vi "WriteOnshapeAngle.vi"(8 "Angle2In":dbl, 9 "Angle1In":dbl, 10 "IDs":T1={"did"="37b1ffe826404682316d4eb0", "wid"="5d55043850c7dcf86f882f4b", "eid"="763f42ab39165e5d749d00a9"}) -> ()   [LabVIEW 2022 SP3]
uses:
  _SubVI/HTTPComm.ctl
panel:
  in  "error in":errorcluster
  out "error out":errorcluster
  out "payload":string
  out "Comm":T2={"url"="https://rogers.onshape.com/api/partstudios/d/78f5bf641b1754cc5a2885a6/w/2816a0ac3f158e698c5324a2/e/990ec2d1208dce12e8c8d73d/sketches?", "sent headers"="Accept: application/json\r\nAuthorization: On 5WRzTWmAmwc94xTxHfKZAg5i:HmacSHA256:lDyQC1x2JlGNCtdzVGE5L8N41PUpGQIlxBBiesg5jjs=\r\nContent-Type: application/json\r\nDate: Thu, 16 Apr 2020 23:19:12 GMT\r\nOn-Nonce: nlS7Y9rr4jS35A8DK9B3OToU\r\nUser_agent: Onshape Python Sample App", "sent body"="", "headers"="HTTP/1.1 200 OK\r\nServer: nginx\r\nDate: Thu, 16 Apr 2020 23:19:12 GMT\r\nContent-Type: application/json;charset=UTF-8;qs=0.9\r\nContent-Length: 2372\r\nConnection: keep-alive\r\nVary: Accept-Encoding\r\nOn-Version: 1.111.25149.0c1f2eb083aa\r\nOn-Request-Id: a78cc699fde7b461387b36e3\r\nDeprecation: version=UNDEFINED, message=\"You specified mediatype application/json;charset=UTF-8;qs=0.9 and this endpoint will currently accept application/vnd.onshape.v1+json;charset=UTF-8;qs=0.1. Please consider updating to the latest version by specifying application/vnd.onshape.v1+json;charset=UTF-8;qs=0.1 within the Accept header.\r\nSet-Cookie: _u=webservice-3e25a82e; Path=/; Secure; HttpOnly;\r\nX-Frame-Options: SAMEORIGIN\r\nStrict-Transport-Security: max-age=31536000; includeSubDomains\r\nX-Content-Type-Options: nosniff\r\nX-XSS-Protection: 1; mode=block\r\nContent-Security-Policy-Report-Only: object-src 'self' https://embedwistia-a.akamaihd.net; report-uri /api/csp\r\n\r\n", "body"="{\n  \"sketches\" : [ {\n    \"sketch\" : \"Sketch 1\",\n    \"featureId\" : \"FbqM6rYzUBbMRp8_0\",\n    \"transformMatrix\" : [ 1.0, 0.0, 0.0, 0.0, 0.0, 1.0, 0.0, 0.0, 0.0, 0.0, 1.0, 0.0, 0.0, 0.0, 0.0, 1.0 ],\n    \"featuresUsed\" : [ ],\n    \"geomEntities\" : [ {\n      \"id\" : \"C471k0qsEi0Q.start\",\n      \"entityType\" : \"point\",\n      \"point\" : [ 0.017283352091908455, -0.007151731755584478 ]\n    }, {\n      \"id\" : \"C471k0qsEi0Q.end\",\n      \"entityType\" : \"point\",\n      \"point\" : [ -0.04529430344700813, 0.05423396825790405 ]\n    }, {\n      \"id\" : \"C471k0qsEi0Q.0.internal\",\n      \"entityType\" : \"point\",\n      \"point\" : [ 0.017283352091908455, -0.007151731755584478 ]\n    }, {\n      \"id\" : \"C471k0qsEi0Q.1.internal\",\n      \"entityType\" : \"point\",\n      \"point\" : [ 0.05095608904957771, 0.022945139557123184 ]\n    }, {\n      \"id\" : \"C471k0qsEi0Q.2.internal\",\n      \"entityType\" : \"point\",\n      \"point\" : [ 0.02443508431315422, 0.05780983343720436 ]\n    }, {\n      \"id\" : \"C471k0qsEi0Q.3.internal\",\n      \"entityType\" : \"point\",\n      \"point\" : [ -0.018177319318056107, 0.039334528148174286 ]\n    }, {\n      \"id\" : \"C471k0qsEi0Q.4.internal\",\n      \"entityType\" : \"point\",\n      \"point\" : [ -0.04529430344700813, 0.05423396825790405 ]\n    }, {\n      \"id\" : \"C471k0qsEi0Q.startDerivative\",\n      \"entityType\" : \"point\",\n      \"point\" : [ 0.03353424071398461, 8.902966705931049E-4 ],\n      \"isConstruction\" : true\n    }, {\n      \"id\" : \"C471k0qsEi0Q.endDerivative\",\n      \"entityType\" : \"point\",\n      \"point\" : [ -0.0368764138795279, 0.04584760236142172 ],\n      \"isConstruction\" : true\n    }, {\n      \"id\" : \"C471k0qsEi0Q\",\n      \"entityType\" : \"interpolatedSplineSegment\",\n      \"periodic\" : false,\n      \"startHandle\" : [ 0.03353424071398461, 8.902966705931043E-4 ],\n      \"endHandle\" : [ -0.03687641387952791, 0.045847602361421734 ],\n      \"startDerivative\" : [ 0.18655982097041743, 0.0923222980796617 ],\n      \"endDerivative\" : [ -0.1167534466674709, 0.11631622339302505 ],\n      \"interpolationPoints\" : [ [ 0.017283352091908455, -0.007151731755584478 ], [ 0.05095608904957771, 0.022945139557123184 ], [ 0.02443508431315422, 0.05780983343720436 ], [ -0.018177319318056107, 0.039334528148174286 ], [ -0.04529430344700813, 0.05423396825790405 ] ],\n      \"startParameter\" : 0.0,\n      \"endParameter\" : 1.0,\n      \"endPointIds\" : [ \"C471k0qsEi0Q.start\", \"C471k0qsEi0Q.end\" ]\n    } ]\n  } ]\n}", "Sent"="get https://rogers.onshape.com/api/partstudios/d/78f5bf641b1754cc5a2885a6/w/2816a0ac3f158e698c5324a2/e/990ec2d1208dce12e8c8d73d/sketches? \n\nAccept: application/json\r\nAuthorization: On 5WRzTWmAmwc94xTxHfKZAg5i:HmacSHA256:lDyQC1x2JlGNCtdzVGE5L8N41PUpGQIlxBBiesg5jjs=\r\nContent-Type: application/json\r\nDate: Thu, 16 Apr 2020 23:19:12 GMT\r\nOn-Nonce: nlS7Y9rr4jS35A8DK9B3OToU\r\nUser_agent: Onshape Python Sample App\n\n", "Received"="HTTP/1.1 200 OK\r\nServer: nginx\r\nDate: Thu, 16 Apr 2020 23:19:12 GMT\r\nContent-Type: application/json;charset=UTF-8;qs=0.9\r\nContent-Length: 2372\r\nConnection: keep-alive\r\nVary: Accept-Encoding\r\nOn-Version: 1.111.25149.0c1f2eb083aa\r\nOn-Request-Id: a78cc699fde7b461387b36e3\r\nDeprecation: version=UNDEFINED, message=\"You specified mediatype application/json;charset=UTF-8;qs=0.9 and this endpoint will currently accept application/vnd.onshape.v1+json;charset=UTF-8;qs=0.1. Please consider updating to the latest version by specifying application/vnd.onshape.v1+json;charset=UTF-8;qs=0.1 within the Accept header.\r\nSet-Cookie: _u=webservice-3e25a82e; Path=/; Secure; HttpOnly;\r\nX-Frame-Options: SAMEORIGIN\r\nStrict-Transport-Security: max-age=31536000; includeSubDomains\r\nX-Content-Type-Options: nosniff\r\nX-XSS-Protection: 1; mode=block\r\nContent-Security-Policy-Report-Only: object-src 'self' https://embedwistia-a.akamaihd.net; report-uri /api/csp\r\n\r\n\n\n{\n  \"sketches\" : [ {\n    \"sketch\" : \"Sketch 1\",\n    \"featureId\" : \"FbqM6rYzUBbMRp8_0\",\n    \"transformMatrix\" : [ 1.0, 0.0, 0.0, 0.0, 0.0, 1.0, 0.0, 0.0, 0.0, 0.0, 1.0, 0.0, 0.0, 0.0, 0.0, 1.0 ],\n    \"featuresUsed\" : [ ],\n    \"geomEntities\" : [ {\n      \"id\" : \"C471k0qsEi0Q.start\",\n      \"entityType\" : \"point\",\n      \"point\" : [ 0.017283352091908455, -0.007151731755584478 ]\n    }, {\n      \"id\" : \"C471k0qsEi0Q.end\",\n      \"entityType\" : \"point\",\n      \"point\" : [ -0.04529430344700813, 0.05423396825790405 ]\n    }, {\n      \"id\" : \"C471k0qsEi0Q.0.internal\",\n      \"entityType\" : \"point\",\n      \"point\" : [ 0.017283352091908455, -0.007151731755584478 ]\n    }, {\n      \"id\" : \"C471k0qsEi0Q.1.internal\",\n      \"entityType\" : \"point\",\n      \"point\" : [ 0.05095608904957771, 0.022945139557123184 ]\n    }, {\n      \"id\" : \"C471k0qsEi0Q.2.internal\",\n      \"entityType\" : \"point\",\n      \"point\" : [ 0.02443508431315422, 0.05780983343720436 ]\n    }, {\n      \"id\" : \"C471k0qsEi0Q.3.internal\",\n      \"entityType\" : \"point\",\n      \"point\" : [ -0.018177319318056107, 0.039334528148174286 ]\n    }, {\n      \"id\" : \"C471k0qsEi0Q.4.internal\",\n      \"entityType\" : \"point\",\n      \"point\" : [ -0.04529430344700813, 0.05423396825790405 ]\n    }, {\n      \"id\" : \"C471k0qsEi0Q.startDerivative\",\n      \"entityType\" : \"point\",\n      \"point\" : [ 0.03353424071398461, 8.902966705931049E-4 ],\n      \"isConstruction\" : true\n    }, {\n      \"id\" : \"C471k0qsEi0Q.endDerivative\",\n      \"entityType\" : \"point\",\n      \"point\" : [ -0.0368764138795279, 0.04584760236142172 ],\n      \"isConstruction\" : true\n    }, {\n      \"id\" : \"C471k0qsEi0Q\",\n      \"entityType\" : \"interpolatedSplineSegment\",\n      \"periodic\" : false,\n      \"startHandle\" : [ 0.03353424071398461, 8.902966705931043E-4 ],\n      \"endHandle\" : [ -0.03687641387952791, 0.045847602361421734 ],\n      \"startDerivative\" : [ 0.18655982097041743, 0.0923222980796617 ],\n      \"endDerivative\" : [ -0.1167534466674709, 0.11631622339302505 ],\n      \"interpolationPoints\" : [ [ 0.017283352091908455, -0.007151731755584478 ], [ 0.05095608904957771, 0.022945139557123184 ], [ 0.02443508431315422, 0.05780983343720436 ], [ -0.018177319318056107, 0.039334528148174286 ], [ -0.04529430344700813, 0.05423396825790405 ] ],\n      \"startParameter\" : 0.0,\n      \"endParameter\" : 1.0,\n      \"endPointIds\" : [ \"C471k0qsEi0Q.start\", \"C471k0qsEi0Q.end\" ]\n    } ]\n  } ]\n}"}
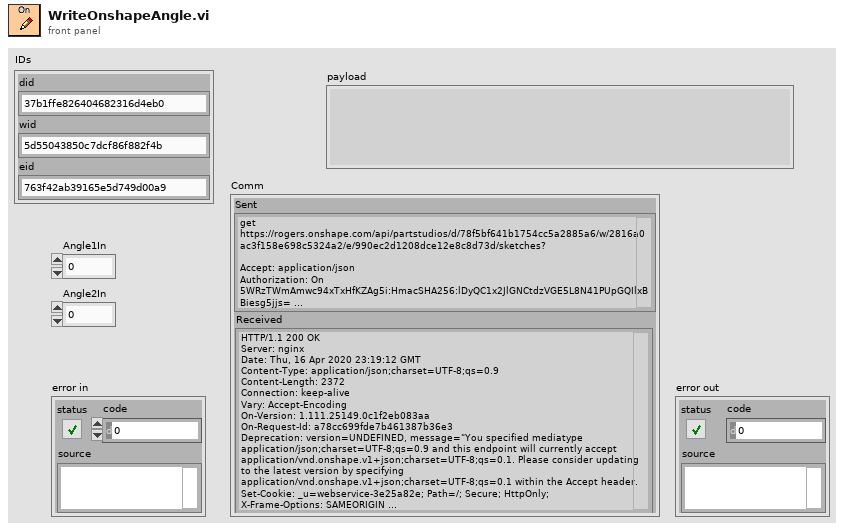
[diagram p1: front panel]
types:
  T1 = cluster{"did":string, "wid":string, "eid":string}
  T2 = typedef "HTTPComm.ctl" = cluster{"url":string, "sent headers":string, "sent body":string, "headers":string, "body":string, "Sent":string, "Received":string}
  T3 = cluster{"mateValues":cluster{"jsonType":string, "rotationZ":dbl, "mateName":string, "featureId":string}[]}
  T4 = cluster{"jsonType":string, "rotationZ":dbl, "mateName":string, "featureId":string}[]
  T5 = cluster{"jsonType":string, "rotationZ":dbl, "mateName":string, "featureId":string}
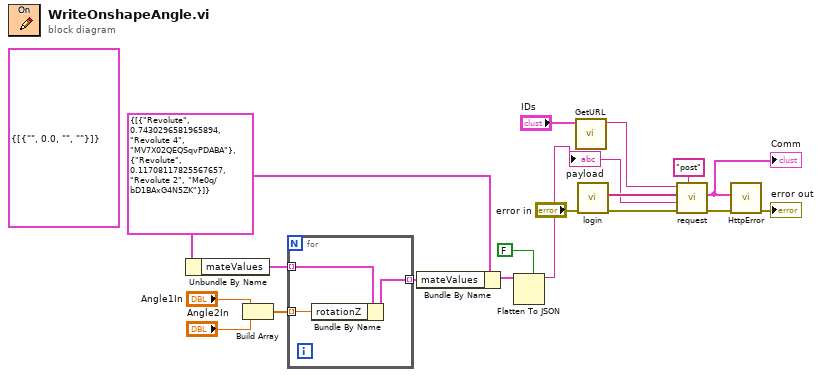
[diagram p0: block diagram]
diagram:
  w5 = T3 {"mateValues"=[{"jsonType"="Revolute", "rotationZ"=0.7430296581965894, "mateName"="Revolute 4", "featureId"="MV7X02QEQSqvPDABA"}, {"jsonType"="Revolute", "rotationZ"=0.11708117825567657, "mateName"="Revolute 2", "featureId"="Me0q/bD1BAxG4N5ZK"}]} ("value")
  (unwired) T3 {"mateValues"=[{"jsonType"="", "rotationZ"=0.0, "mateName"="", "featureId"=""}]}
  n1 = Unbundle By Name(w5) -> ("mateValues"=w9:T4)
  n2 = Build Array("Angle1In", "Angle2In") -> (w6:dbl[])
  n3 = for {
    tunnel: w9 -> [w21] mode=indexing
    tunnel: w6 -> [w20] mode=indexing
    tunnel: [w19] -> w4 mode=indexing
    n4 = Bundle By Name(cluster=w21, "rotationZ"=w20) -> (w19:T5)
  }
  n5 = Bundle By Name(cluster=w5, "mateValues"=w4) -> (w3:T3)
  n6 = Flatten To JSON(enable LabVIEW extensions? (T)=FALSE, anything=w3) -> (JSON string=w1:string)  [unwired: 1 in, 1 out]
  "payload" <- w1
  n7 = call "GetURL.vi"("IDs"="IDs") -> ("String"=w13:string)  [unwired: 10 in]
  n8 = call "login.vi"("error in"="error in") -> ("error out"=w16:errorcluster, "Headers"=w17:string[])  [unwired: 9 in]
  n9 = call "request.vi"("URL"=w13, "headers"=w17, "POST Payload"=w1, "error in"=w16, "method"="post" ("Method")) -> ("Comm"=w12:T2, "error out"=w14:errorcluster)  [unwired: 4 in]
  "Comm" <- w12
  n10 = call "HttpError.vi"("error in (no error)"=w14, "Comm"=w12) -> ("error out"=→"error out":errorcluster)  [unwired: 8 in, 1 out]
